vi "Teleop.vi"(10 "Match Info":T1={"Autonomous Elapsed Seconds"=0.0, "TeleOp Elapsed Seconds"=0.0, "Disabled Elapsed Seconds"=0.0, "Visited Autonomous"=FALSE, "Visited TeleOp"=FALSE, "Visited Disabled"=FALSE, "Autonomous Settings"={"Autonomous Style"=enum."Independent", "VI Refnum"=refnum}}, 11 "Call Context":T2) -> ()   [LabVIEW 2018]
doc: "This VI is called for each enabled TeleOp packet received from the DS. It is typically used to read from joysticks and other inputs and update I/O or setpoints for timed control loops. It should complete and return within 20 milliseconds or risk missing DS packets."
uses:
  <vilib>/Rock Robotics/WPI/DriverStation/WPI_DriverStationDerivedRobotMode.ctl
  <vilib>/Rock Robotics/WPI/DriverStation/WPI_DriverStationMatch Info.ctl
  <vilib>/Rock Robotics/WPI/ThirdParty/Phoenix-LabVIEW/Motor Controller/Controls/CTRE_Phoenix_MotorControl_ControlMode.ctl
  2fc8d68a-f7f1-41dc-b85b-aa47af0e09c4.vi
  <vilib>/Rock Robotics/WPI/Utilities/WPI_GetSetVariantRefNum.vi
  <vilib>/Rock Robotics/Network Tables/NT Write Boolean.vi
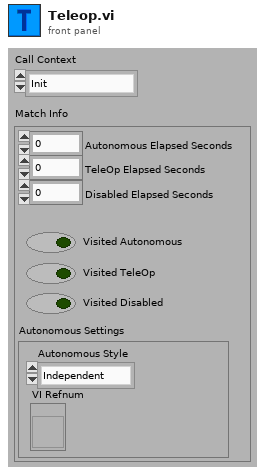
[diagram p1: front panel]
types:
  T1 = typedef "WPI_DriverStationMatch Info.ctl" = cluster{"Autonomous Elapsed Seconds":dbl, "TeleOp Elapsed Seconds":dbl, "Disabled Elapsed Seconds":dbl, "Visited Autonomous":bool, "Visited TeleOp":bool, "Visited Disabled":bool, "Autonomous Settings":cluster{"Autonomous Style":enum16{"Iterative", "Independent"}, "VI Refnum":refnum<vi>}}
  T2 = typedef "WPI_DriverStationDerivedRobotMode.ctl" = enum16{"Init", "Execute", "Stop"}
  T3 = enum16{"Low Ball", "Middle Ball", "High Ball", "High Hatch", "Middle Hatch", "Low Hatch", "Cargo Ball", "Ball Loading Station", "Ball Ground", "Reserve"}
  T4 = typedef "WPI_JoystickDevRef.ctl" = cluster{"Device":T5}
  T5 = typedef "WPI_JoystickDeviceEnum.ctl" = enum16{"USB 0", "USB 1", "USB 2", "USB 3", "USB 4", "USB 5"}
  T6 = cluster{"POVs[0]":i16, "POVs[1]":i16, "POVs[2]":i16, "POVs[3]":i16, "POVs[4]":i16, "POVs[5]":i16, "POVs[6]":i16, "POVs[7]":i16, "POVs[8]":i16}
  T7 = typedef "WPI_MotorControlDeviceRef.ctl" = cluster{"DeviceStatus":errorcluster, "Type":T8, "PWM":cluster{"PWM Channel":T9, "DeadBand":T10}, "CAN":cluster{"Device Number":u8, "SetOutput VI Ref":variant, "GetOutput VI Ref":variant, "Enable VI Ref":variant, "Disable VI Ref":variant, "Data":variant}, "Invert":bool, "DIO PWM":cluster{"PWM \"Enable\" Channel":T9, "DIOChannel":T11, "PWM Rate":dbl}}
  T8 = typedef "WPI_MotorControlType.ctl" = enum16{"PWM", "CAN", "DIO PWM"}
  T9 = typedef "FPGA_DIOPWMChannel.ctl" = enum8{"PWM 0", "PWM 1", "PWM 2", "PWM 3", "PWM 4", "PWM 5", "PWM 6", "PWM 7", "PWM 8", "PWM 9", "PWM MXP 0", "PWM MXP 1", "PWM MXP 2", "PWM MXP 3", "PWM MXP 4", "PWM MXP 5", "PWM MXP 6", "PWM MXP 7", "PWM MXP 8", "PWM MXP 9", "Invalid"}
  T10 = typedef "WPI_PWMDeadband.ctl" = cluster{"Name":string, "maxPositivePwm":i32, "minPositivePwm":i32, "centerPwm":i32, "maxNegativePwm":i32, "minNegativePwm":i32, "angularRange":u16}
  T11 = typedef "FPGA_DIOChannel.ctl" = enum8{"DIO 0", "DIO 1", "DIO 2", "DIO 3", "DIO 4", "DIO 5", "DIO 6", "DIO 7", "DIO 8", "DIO 9", "DIO MXP 0", "DIO MXP 1", "DIO MXP 2", "DIO MXP 3", "DIO MXP 4", "DIO MXP 5", "DIO MXP 6", "DIO MXP 7", "DIO MXP 8", "DIO MXP 9", "DIO MXP 10", "DIO MXP 11", "DIO MXP 12", "DIO MXP 13", "DIO MXP 14", "DIO MXP 15", "SPI Port CS1", "SPI Port CS2", "SPI Port CS3", "SPI Port MISO", "SPI Port MOSI", "Invalid"}
  T12 = typedef "CTRE_Phoenix_MotorControl_ControlMode.ctl" = u16
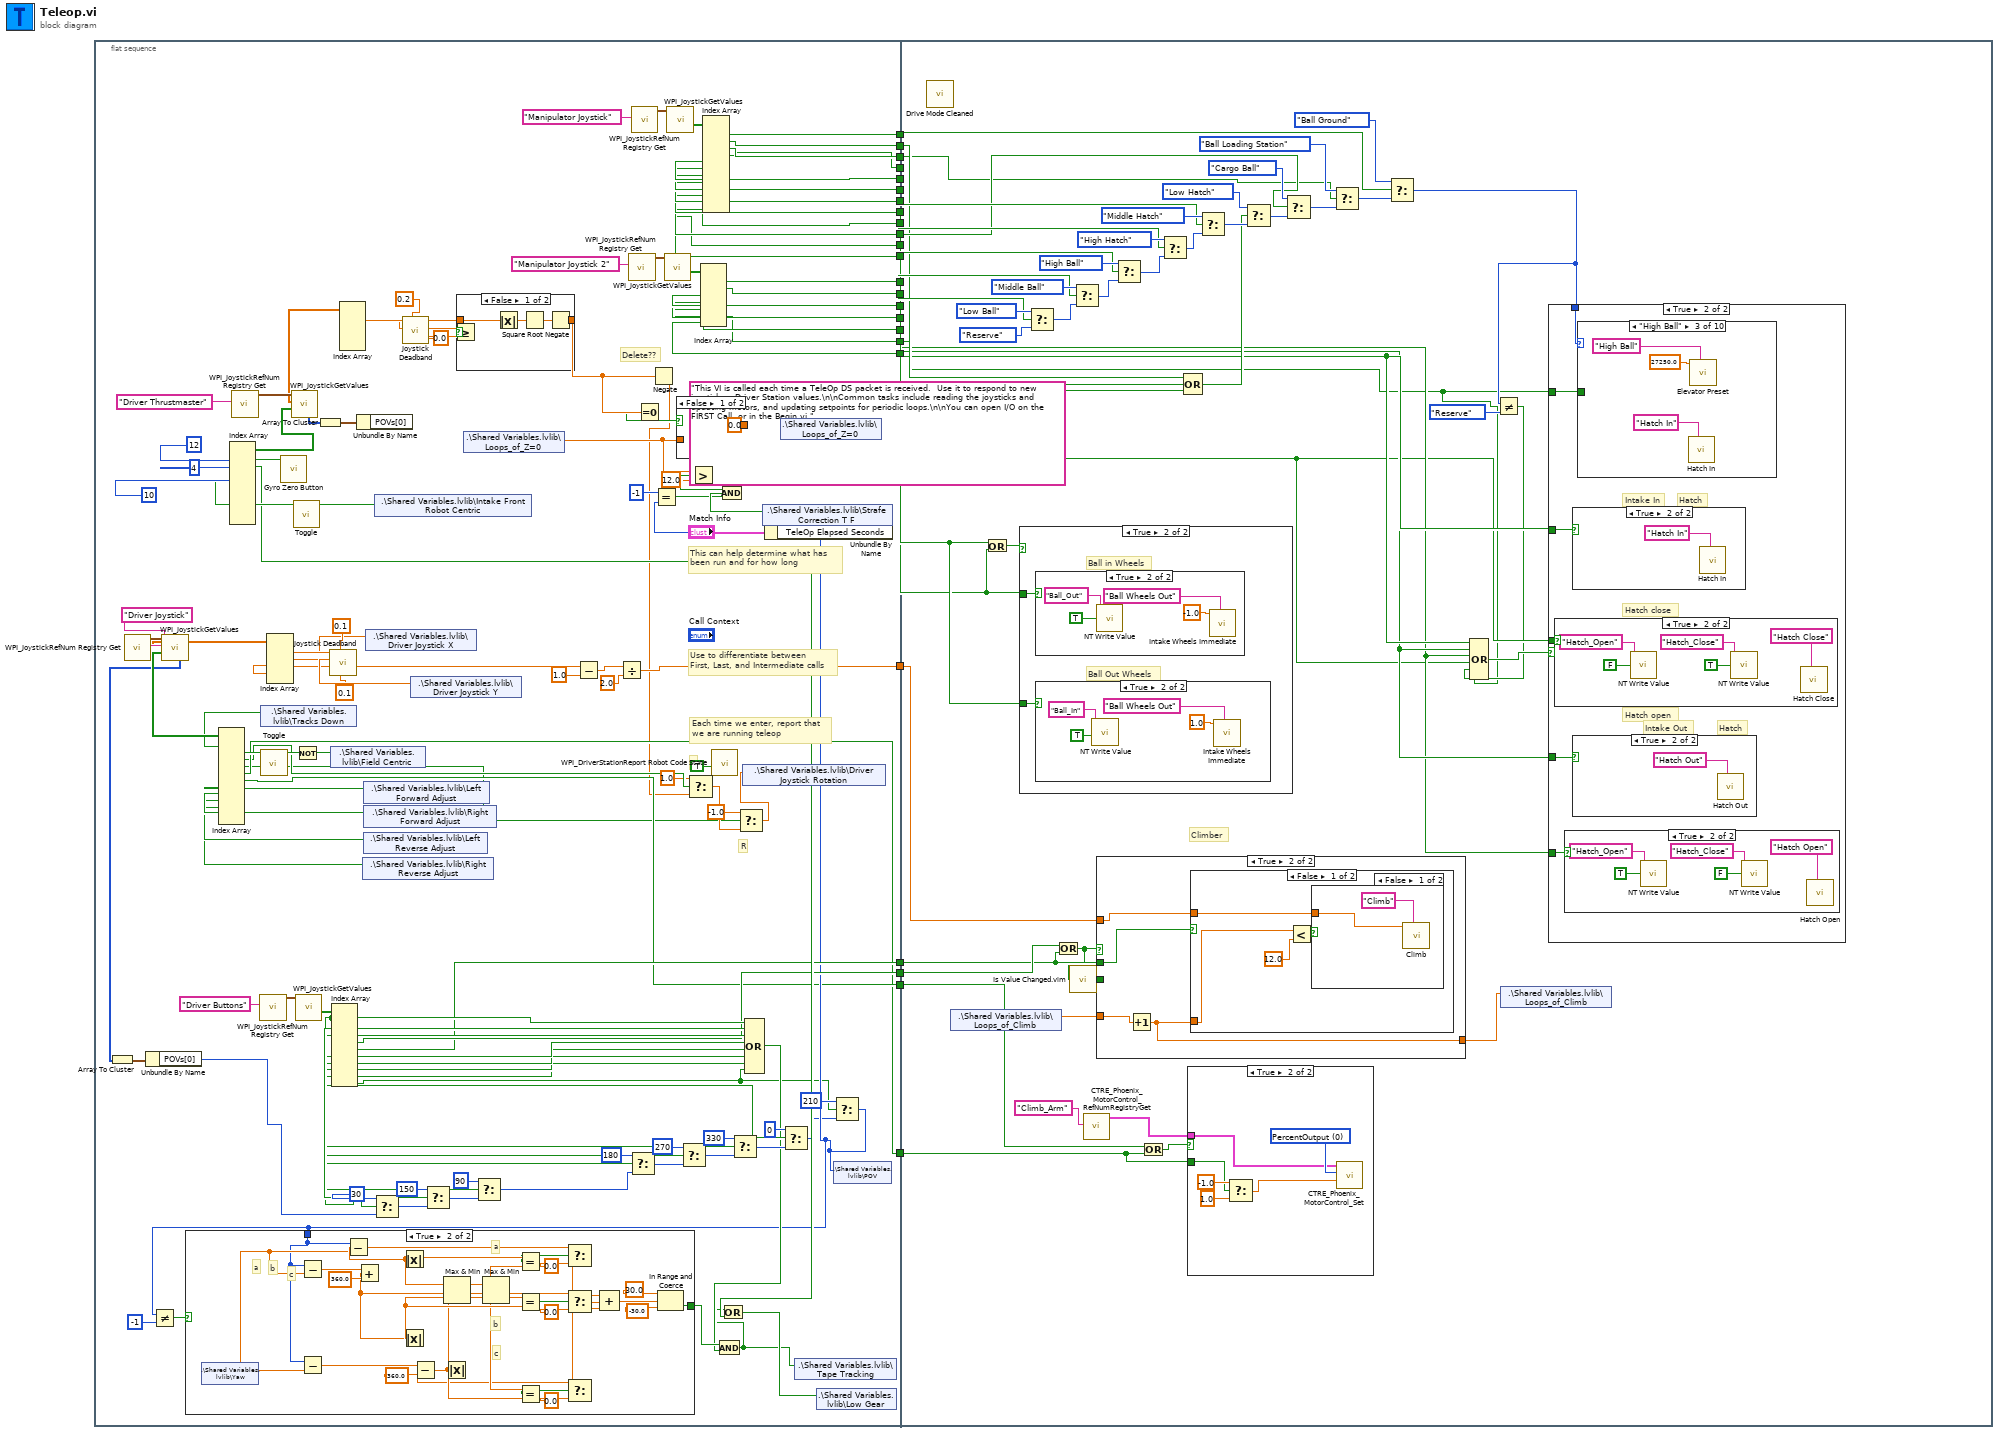
[diagram p0: block diagram]
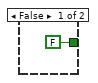
[diagram p2: hidden frame]
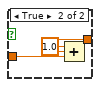
[diagram p3: hidden frame]
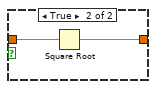
[diagram p4: hidden frame]
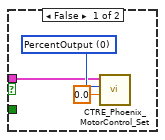
[diagram p5: hidden frame]
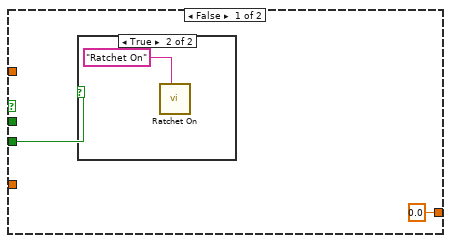
[diagram p6: hidden frame]
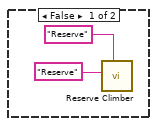
[diagram p7: hidden frame]
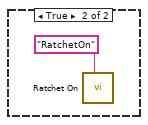
[diagram p8: hidden frame]
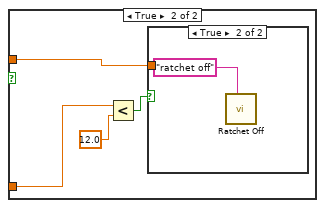
[diagram p9: hidden frame]
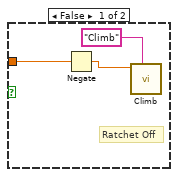
[diagram p10: hidden frame]
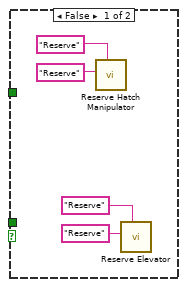
[diagram p11: hidden frame]
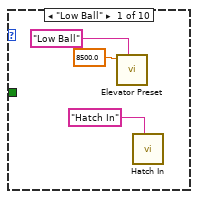
[diagram p12: hidden frame]
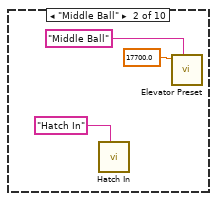
[diagram p13: hidden frame]
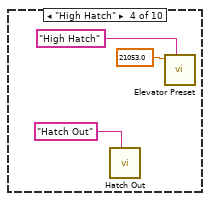
[diagram p14: hidden frame]
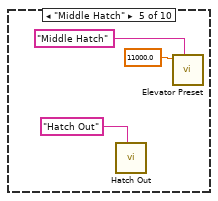
[diagram p15: hidden frame]
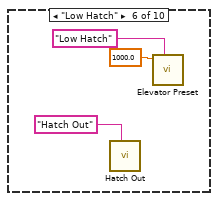
[diagram p16: hidden frame]
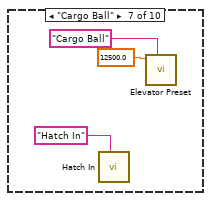
[diagram p17: hidden frame]
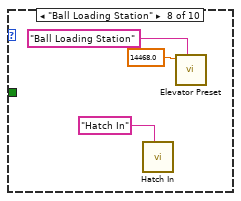
[diagram p18: hidden frame]
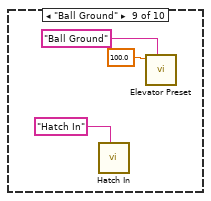
[diagram p19: hidden frame]
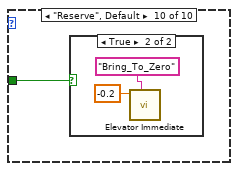
[diagram p20: hidden frame]
diagram:
  (unwired) "This VI is called each time a TeleOp DS packet is received.  Use it to respond to new joystick or Driver Station values.\n\nCommon tasks include reading the joysticks and updating motors, and updating setpoints for periodic loops.\n\nYou can open I/O on the FIRST Call, or in the Begin.vi."
  # "Each time we enter, report that\nwe are running teleop"
  # "Use to differentiate between\nFirst, Last, and Intermediate calls"
  # "This can help determine what has\nbeen run and for how long"
  n1 = flat-sequence {
    tunnel: [w50] -> w24
    tunnel: [w108] -> w23
    tunnel: [w107] -> w22
    tunnel: [w106] -> w21
    tunnel: [w105] -> w20
    tunnel: [w104] -> w19
    tunnel: [w103] -> w18
    tunnel: [w102] -> w17
    tunnel: [w101] -> w16
    tunnel: [w100] -> w15
    tunnel: [w99] -> w14
    tunnel: [w98] -> w13
    tunnel: [w97] -> w12
    tunnel: [w96] -> w11
    tunnel: [w95] -> w10
    tunnel: [w94] -> w9
    tunnel: [w93] -> w8
    tunnel: [w92] -> w7
    tunnel: [w91] -> w6
    tunnel: [w90] -> w5
    tunnel: [w53] -> w4
    tunnel: [w52] -> w3
    tunnel: [w36] -> w2
    tunnel: [w34] -> w1
    tunnel: w24 -> [w199]
    tunnel: w23 -> [w214]
    tunnel: w22 -> [w217]
    tunnel: w21 -> [w213]
    tunnel: w20 -> [w219]
    tunnel: w19 -> [w216]
    tunnel: w18 -> [w222]
    tunnel: w17 -> [w220]
    tunnel: w16 -> [w209]
    tunnel: w15 -> [w223]
    tunnel: w14 -> [w218]
    tunnel: w13 -> [w221]
    tunnel: w12 -> [w210]
    tunnel: w11 -> [w205]
    tunnel: w10 -> [_]
    tunnel: w9 -> [w208]
    tunnel: w8 -> [w206]
    tunnel: w7 -> [w207]
    tunnel: w6 -> [w197]
    tunnel: w5 -> [w212]
    tunnel: w4 -> [w201]
    tunnel: w3 -> [w200]
    tunnel: w2 -> [w193]
    tunnel: w1 -> [w192]
    frame #0 {
      # "R"
      # "L"
      # "Delete??"
      n2 = call <vilib>:"WPI_JoystickRefNum Registry Get.vi"("refnum name"="Driver Joystick") -> ("JoystickDevRef"=w149:T4)  [unwired: 1 in, 9 out]
      n3 = call <vilib>:"WPI_JoystickGetValues.vi"("JoystickDevRef"=w149) -> ("Buttons"=w135:bool[], "Axes"=w147:dbl[], "POVs"=w122:i16[])  [unwired: 6 in, 2 out]
      n4 = Array To Cluster(array=w122) -> (cluster=w123:T6)
      n5 = Unbundle By Name(w123) -> ("POVs[0]"=w35:i16)
      n6 = Index Array(array=w135) -> (element #1=w111:bool, element #2=w110:bool, element #3=w33:bool, element #4=w31:bool, element #5=w34:bool, element #6=w36:bool, element #7=w120:bool, element #8=w119:bool, element #9=w118:bool, element #10=w117:bool)  [unwired: 12 in, 2 out]
      n7 = call <vilib>:"WPI_JoystickRefNum Registry Get.vi"("refnum name"="Driver Thrustmaster") -> ("JoystickDevRef"=w137:T4)  [unwired: 9 in, 1 out]
      n8 = call <vilib>:"WPI_JoystickRefNum Registry Get.vi"("refnum name"="Driver Buttons") -> ("JoystickDevRef"=w88:T4)  [unwired: 1 in, 9 out]
      n9 = shared-variable ".\\Shared Variables.lvlib\\Tracks Down"(w111) -> ()  [unwired: 1 in, 1 out]
      n10 = call "Toggle.vi"("Input"=w110) -> ("Output"=w142:bool)  [unwired: 9 in, 1 out]
      n11 = Index Array(array=w147) -> (element #1=w141:dbl, element #2=w140:dbl, element #4=w112:dbl)  [unwired: 5 in, 2 out]
      n12 = call <vilib>:"WPI_JoystickGetValues.vi"("JoystickDevRef"=w137) -> ("Buttons"=w132:bool[], "Axes"=w136:dbl[], "POVs"=w124:i16[])  [unwired: 6 in, 2 out]
      n13 = Index Array(array=w132, index #1=12 ("index"), index #2=4 ("index"), index #4=10 ("index")) -> (element #1=w130:bool, element #2=w56:bool, element #4=w125:bool)  [unwired: 7 in, 7 out]
      n14 = call "Gyro Zero Button.vi"("Boolean"=w130) -> ()  [unwired: 11 in]
      n15 = call "Toggle.vi"("Input"=w125) -> ("Output"=w126:bool)  [unwired: 9 in, 1 out]
      n16 = Not(x=w142) -> (.not. x?=w139:bool)
      n17 = call <vilib>:"WPI_JoystickGetValues.vi"("JoystickDevRef"=w88) -> ("Buttons"=w48:bool[])  [unwired: 6 in, 4 out]
      n18 = Array To Cluster(array=w124) -> (cluster=w128:T6)
      n19 = call "Joystick Deadband.vi"("Z Deadband"=0.1, "X Y Deadband"=0.1, "Z"=w112, "Y"=w140, "X"=w141) -> ("Z Out"=w39:dbl, "Y Out"=w143:dbl, "X Out"=w116:dbl)  [unwired: 4 in]
      n20 = shared-variable ".\\Shared Variables.lvlib\\Field Centric"(w139) -> ()  [unwired: 1 in, 1 out]
      n21 = Index Array(array=w48) -> (element #1=w68:bool, element #2=w74:bool, element #3=w73:bool, element #4=w53:bool, element #5=w52:bool, element #6=w72:bool, element #7=w71:bool, element #8=w70:bool, element #9=w69:bool, element #10=w40:bool)  [unwired: 10 in]
      n22 = Index Array(array=w136) -> (element #1=w115:dbl)  [unwired: 5 in, 4 out]
      n23 = Unbundle By Name(w128) -> ()  [unwired: 1 out]
      n24 = shared-variable ".\\Shared Variables.lvlib\\Right Reverse Adjust"(w117) -> ()  [unwired: 1 in, 1 out]
      n25 = shared-variable ".\\Shared Variables.lvlib\\Left Forward Adjust"(w120) -> ()  [unwired: 1 in, 1 out]
      n26 = shared-variable ".\\Shared Variables.lvlib\\Right Forward Adjust"(w119) -> ()  [unwired: 1 in, 1 out]
      n27 = shared-variable ".\\Shared Variables.lvlib\\Left Reverse Adjust"(w118) -> ()  [unwired: 1 in, 1 out]
      n28 = shared-variable ".\\Shared Variables.lvlib\\Driver Joystick X"(w116) -> ()  [unwired: 1 in, 1 out]
      n29 = Select(t=i16 30, s=w68, f=w35) -> (s? t:f=w82:i16)
      n30 = shared-variable ".\\Shared Variables.lvlib\\Intake Front Robot Centric"(w126) -> ()  [unwired: 1 in, 1 out]
      n31 = call "Joystick Deadband.vi"("X Y Deadband"=0.2, "X"=w115) -> ("X Out"=w113:dbl)  [unwired: 7 in, 2 out]
      n32 = shared-variable ".\\Shared Variables.lvlib\\Driver Joystick Y"(w143) -> ()  [unwired: 1 in, 1 out]
      n33 = Select(t=i16 150, s=w74, f=w82) -> (s? t:f=w81:i16)
      n34 = Greater Or Equal?(x=w113, y=0.0) -> (x >= y?=w134:bool)
      n35 = case shown="False" w134 {
        tunnel: [w183 w187] -> w64
        tunnel: w113 -> [w182 w186]
        frame False {
          n36 = Absolute Value(x=w182) -> (abs(x)=w185:dbl)
          n37 = Square Root(x=w185) -> (sqrt(x)=w184:dbl)
          n38 = Negate(x=w184) -> (-x=w183:dbl)
        }
        frame True {
          n39 = Square Root(x=w186) -> (sqrt(x)=w187:dbl)
        }
      }
      n40 = shared-variable ".\\Shared Variables.lvlib\\Loops_of_Z=0"() -> (w60:dbl)  [unwired: 1 in, 1 out]
      n41 = Select(t=i16 90, s=w73, f=w81) -> (s? t:f=w49:i16)
      n42 = Subtract(x=w39, y=1.0) -> (x-y=w38:dbl)
      n43 = Divide(x=w38, y=2.0) -> (x/y=w50:dbl)
      n44 = call <vilib>:"WPI_JoystickRefNum Registry Get.vi"("refnum name"="Manipulator Joystick 2") -> ("JoystickDevRef"=w89:T4)  [unwired: 1 in, 9 out]
      n45 = Select(t=i16 180, s=w72, f=w49) -> (s? t:f=w79:i16)
      n46 = call <vilib>:"WPI_JoystickRefNum Registry Get.vi"("refnum name"="Manipulator Joystick") -> ("JoystickDevRef"=w145:T4)  [unwired: 1 in, 9 out]
      n47 = Equal To 0?(x=w64) -> (x = 0?=w63:bool)
      n48 = Negate(x=w64) -> (-x=w28:dbl)
      n49 = call <vilib>:"WPI_JoystickGetValues.vi"("JoystickDevRef"=w89) -> ("Buttons"=w46:bool[])  [unwired: 6 in, 4 out]
      n50 = call <vilib>:"WPI_JoystickGetValues.vi"("JoystickDevRef"=w145) -> ("Buttons"=w47:bool[])  [unwired: 6 in, 4 out]
      n51 = case shown="False" w63 {
        tunnel: w60 -> [_ w181]
        tunnel: [0.0 w179] -> w62
        frame False {
        }
        frame True {
          n52 = Add(x=1.0, y=w181) -> (x+y=w179:dbl)
        }
      }
      n53 = Select(t=i16 270, s=w71, f=w79) -> (s? t:f=w77:i16)
      n54 = Select(t=1.0, s=w33, f=w28) -> (s? t:f=w32:dbl)
      n55 = Greater?(x=w60, y=12.0) -> (0:w61:bool)
      n56 = Index Array(array=w46) -> (element #1=w96:bool, element #2=w95:bool, element #3=w94:bool, element #4=w93:bool, element #5=w92:bool, element #6=w91:bool, element #7=w90:bool)  [unwired: 7 in]
      n57 = Index Array(array=w47) -> (element #1=w108:bool, element #2=w107:bool, element #3=w106:bool, element #4=w105:bool, element #5=w104:bool, element #6=w103:bool, element #7=w102:bool, element #8=w101:bool, element #9=w100:bool, element #10=w99:bool, element #11=w98:bool, element #12=w97:bool)  [unwired: 12 in]
      n58 = Select(t=i16 330, s=w70, f=w77) -> (s? t:f=w75:i16)
      n59 = Select(t=-1.0, s=w31, f=w32) -> (s? t:f=w27:dbl)
      n60 = shared-variable ".\\Shared Variables.lvlib\\Driver Joystick Rotation"(w27) -> ()  [unwired: 1 in, 1 out]
      n61 = Compound Arithmetic op=OR(w68, w74, w73, w72, w71, w70, w69, w40) -> (w57:bool)
      n62 = shared-variable ".\\Shared Variables.lvlib\\Loops_of_Z=0"(w62) -> ()  [unwired: 1 in, 1 out]
      n63 = Select(t=i16 0, s=w69, f=w75) -> (s? t:f=w42:i16)
      n64 = Select(t=i16 210, s=w40, f=w42) -> (s? t:f=w43:i16)
      n65 = Not Equal?(x=w43, y=i16 -1) -> (x != y?=w45:bool)
      n66 = case shown="True" w45 {
        tunnel: [FALSE w175] -> w58
        tunnel: w43 -> [_ w152]
        frame False {
        }
        frame True {
          # "c"
          # "b"
          # "a"
          # "c"
          # "b"
          # "a"
          n67 = shared-variable ".\\Shared Variables.lvlib\\Yaw"() -> (w153:dbl)  [unwired: 1 in, 1 out]
          n68 = Subtract(x=w152, y=w153) -> (x-y=w174:dbl)
          n69 = Subtract(x=w152, y=w153) -> (x-y=w172:dbl)
          n70 = Subtract(x=w152, y=w153) -> (x-y=w163:dbl)
          n71 = Add(x=w174, y=360.0) -> (x+y=w164:dbl)
          n72 = Absolute Value(x=w163) -> (abs(x)=w169:dbl)
          n73 = Absolute Value(x=w164) -> (abs(x)=w168:dbl)
          n74 = Subtract(x=w172, y=360.0) -> (x-y=w162:dbl)
          n75 = Max & Min(x=w169, y=w168) -> (min(x,y)=w170:dbl)  [unwired: 1 out]
          n76 = Absolute Value(x=w162) -> (abs(x)=w166:dbl)
          n77 = Max & Min(x=w170, y=w166) -> (min(x,y)=w167:dbl)  [unwired: 1 out]
          n78 = Equal?(x=w169, y=w167) -> (x = y?=w161:bool)
          n79 = Equal?(x=w167, y=w168) -> (x = y?=w165:bool)
          n80 = Equal?(x=w167, y=w166) -> (x = y?=w160:bool)
          n81 = Select(t=w163, s=w161, f=0.0) -> (s? t:f=w156:dbl)
          n82 = Select(t=w164, s=w165, f=0.0) -> (s? t:f=w155:dbl)
          n83 = Select(t=w162, s=w160, f=0.0) -> (s? t:f=w154:dbl)
          n84 = Compound Arithmetic op=ADD(w156, w155, w154) -> (w151:dbl)
          n85 = In Range and Coerce(upper limit=30.0, x=w151, lower limit=-30.0) -> (In Range?=w175:bool)  [unwired: 1 out]
        }
      }
      n86 = Equal?(x=i16 -1, y=w43) -> (x = y?=w65:bool)
      n87 = And(x=w61, y=w65) -> (x .and. y?=w66:bool)
      n88 = Compound Arithmetic op=AND(w58, w57) -> (w54:bool)
      n89 = Or(x=w54, y=w56) -> (x .or. y?=w55:bool)
      n90 = shared-variable ".\\Shared Variables.lvlib\\Strafe Correction T F"(w66) -> ()  [unwired: 1 in, 1 out]
      n91 = shared-variable ".\\Shared Variables.lvlib\\Tape Tracking"(w54) -> ()  [unwired: 1 in, 1 out]
      n92 = shared-variable ".\\Shared Variables.lvlib\\Low Gear"(w55) -> ()  [unwired: 1 in, 1 out]
      n93 = shared-variable ".\\Shared Variables.lvlib\\POV"(w43) -> ()  [unwired: 1 in, 1 out]
    }
    frame #1 {
      # "Climber"
      n94 = call "Drive Mode Cleaned.vi"() -> ()  [unwired: 12 in]
      n95 = shared-variable ".\\Shared Variables.lvlib\\Loops_of_Climb"() -> (w189:dbl)  [unwired: 1 in, 1 out]
      n96 = Or(x=w210, y=w209) -> (x .or. y?=w211:bool)
      n97 = case shown="True" w211 {
        tunnel: w210 -> [_ w336]
        tunnel: w209 -> [_ w335]
        frame False {
          n98 = call-poly <vilib>:"NT Write Value.vi"("Boolean"=FALSE, "Name"="Ball_Out") -> ()  [unwired: 9 in, 1 out]
          n99 = call "Reserve Intake.vi"("Description"="Reserve", "Command Name"="Reserve") -> ()  [unwired: 9 in, 1 out]
          n100 = call-poly <vilib>:"NT Write Value.vi"("Boolean"=FALSE, "Name"="Ball_In") -> ()  [unwired: 9 in, 1 out]
        }
        frame True {
          # "Ball in Wheels"
          # "Ball Out Wheels"
          n101 = case shown="True" w335 {
            frame False {
            }
            frame True {
              n102 = call-poly <vilib>:"NT Write Value.vi"("Boolean"=TRUE, "Name"="Ball_Out") -> ()  [unwired: 9 in, 1 out]
              n103 = call "Intake Wheels Immediate.vi"("Description"="Ball Wheels Out", "Setpoint"=-1.0) -> ()  [unwired: 9 in, 1 out]
            }
          }
          n104 = case shown="True" w336 {
            frame False {
            }
            frame True {
              n105 = call-poly <vilib>:"NT Write Value.vi"("Boolean"=TRUE, "Name"="Ball_In") -> ()  [unwired: 9 in, 1 out]
              n106 = call "Intake Wheels Immediate.vi"("Description"="Ball Wheels Out", "Setpoint"=1.0) -> ()  [unwired: 9 in, 1 out]
            }
          }
        }
      }
      n107 = Select(t=T3."Low Ball" ("Enum"), s=w219, f=T3."Reserve" ("Enum")) -> (s? t:f=w241:T3)
      n108 = Or(x=w201, y=w200) -> (x .or. y?=w191:bool)
      n109 = call "Is Value Changed.vim"("value"=w191) -> ("changed or first call?"=w190:bool)
      n110 = Select(t=T3."Middle Ball" ("Enum"), s=w220, f=w241) -> (s? t:f=w240:T3)
      n111 = call <vilib>:"CTRE_Phoenix_MotorControl_RefNumRegistryGet.vi"("refnum name"="Climb_Arm") -> ("PhoenixMotorControlDevRef"=w195:T7)  [unwired: 9 in, 1 out]
      n112 = case shown="True" w191 {
        tunnel: w200 -> [_ w259]
        tunnel: w199 -> [_ w258]
        tunnel: w190 -> [w252 _]
        tunnel: w189 -> [_ w257]
        tunnel: [0.0 w256] -> w188
        frame False {
          n113 = case shown="True" w252 {
            frame False {
              n114 = call "Reserve Climber.vi"("Description"="Reserve", "Command Name"="Reserve" ("Description")) -> ()  [unwired: 9 in, 1 out]
            }
            frame True {
              n115 = call "Ratchet On.vi"("Description"="Ratchet On") -> ()  [unwired: 10 in, 1 out]
            }
          }
        }
        frame True {
          n116 = Increment(x=w257) -> (x+1=w256:dbl)
          n117 = case shown="False" w259 {
            tunnel: w258 -> [w263 w270]
            tunnel: w256 -> [w260 w267]
            frame False {
              n118 = Less?(x=w260, y=12.0 ("x")) -> (x < y?=w262:bool)
              n119 = case shown="False" w262 {
                tunnel: w263 -> [w264 _]
                frame False {
                  n120 = call "Climb.vi"("Description"="Climb", "Setpoint"=w264) -> ()  [unwired: 9 in, 1 out]
                }
                frame True {
                  n121 = call "Ratchet On.vi"("Description"="RatchetOn") -> ()  [unwired: 10 in, 1 out]
                }
              }
            }
            frame True {
              n122 = Less?(x=w267, y=12.0 ("x")) -> (x < y?=w268:bool)
              n123 = case shown="True" w268 {
                tunnel: w270 -> [w272 _]
                frame False {
                  # "Ratchet Off"
                  n124 = Negate(x=w272) -> (-x=w271:dbl)
                  n125 = call "Climb.vi"("Description"="Climb", "Setpoint"=w271) -> ()  [unwired: 9 in, 1 out]
                }
                frame True {
                  n126 = call "Ratchet Off.vi"("Description"="ratchet off") -> ()  [unwired: 10 in, 1 out]
                }
              }
            }
          }
        }
      }
      n127 = Select(t=T3."High Ball" ("Enum"), s=w221, f=w240) -> (s? t:f=w239:T3)
      n128 = Or(x=w193, y=w192) -> (x .or. y?=w194:bool)
      n129 = Select(t=T3."High Hatch" ("Enum"), s=w223, f=w239) -> (s? t:f=w238:T3)
      n130 = Compound Arithmetic op=OR(w217, w216, w212) -> (w215:bool)
      n131 = case shown="True" w194 {
        tunnel: w195 -> [w242 w245]
        tunnel: w192 -> [_ w247]
        frame False {
          w244 = T12 0 items=["PercentOutput"=0, "Position"=1, "Velocity"=2, "Current"=3, "Follower"=5, "MotionProfile"=6, "MotionMagic"=7, "MotionProfileArc"=10, "Disabled"=15] ("Control Mode")
          n132 = call <vilib>:"CTRE_Phoenix_MotorControl_Set.vi"("Output"=0.0, "Control Mode"=w244, "PhoenixMotorControlDevRef"=w242) -> ()  [unwired: 7 in, 2 out]
        }
        frame True {
          w250 = T12 0 items=["PercentOutput"=0, "Position"=1, "Velocity"=2, "Current"=3, "Follower"=5, "MotionProfile"=6, "MotionMagic"=7, "MotionProfileArc"=10, "Disabled"=15] ("Control Mode")
          n133 = Select(t=-1.0, s=w247, f=1.0) -> (s? t:f=w246:dbl)
          n134 = call <vilib>:"CTRE_Phoenix_MotorControl_Set.vi"("Output"=w246, "Control Mode"=w250, "PhoenixMotorControlDevRef"=w245) -> ()  [unwired: 7 in, 2 out]
        }
      }
      n135 = Select(t=T3."Middle Hatch" ("Enum"), s=w222, f=w238) -> (s? t:f=w237:T3)
      n136 = Select(t=T3."Low Hatch" ("Enum"), s=w215, f=w237) -> (s? t:f=w236:T3)
      n137 = Select(t=T3."Cargo Ball" ("Enum"), s=w218, f=w236) -> (s? t:f=w235:T3)
      n138 = Select(t=T3."Ball Loading Station" ("Enum"), s=w213, f=w235) -> (s? t:f=w225:T3)
      n139 = Select(t=T3."Ball Ground" ("Enum"), s=w214, f=w225) -> (s? t:f=w203:T3)
      n140 = Not Equal?(x=w203, y=T3."Reserve" ("Enum")) -> (x != y?=w198:bool)
      n141 = Compound Arithmetic op=OR(w208, w207, w206, w205, w198, w197) -> (w204:bool)
      n142 = shared-variable ".\\Shared Variables.lvlib\\Loops_of_Climb"(w188) -> ()  [unwired: 1 in, 1 out]
      n143 = case shown="True" w204 {
        tunnel: w208 -> [_ w284]
        tunnel: w206 -> [_ w283]
        tunnel: w207 -> [_ w282]
        tunnel: w205 -> [_ w281]
        tunnel: w203 -> [_ w280]
        tunnel: w197 -> [_ w279]
        frame False {
          n144 = call "Reserve Hatch Manipulator.vi"("Description"="Reserve", "Command Name"="Reserve") -> ()  [unwired: 9 in, 1 out]
          n145 = call "Reserve Elevator.vi"("Description"="Reserve", "Command Name"="Reserve") -> ()  [unwired: 9 in, 1 out]
        }
        frame True {
          # "Hatch"
          # "Hatch"
          # "Hatch open"
          # "Hatch close"
          # "Intake In"
          # "Intake Out"
          n146 = case shown="True" w281 {
            frame False {
            }
            frame True {
              n147 = call-poly <vilib>:"NT Write Value.vi"("Boolean"=FALSE, "Name"="Hatch_Open") -> ()  [unwired: 9 in, 1 out]
              n148 = call-poly <vilib>:"NT Write Value.vi"("Boolean"=TRUE, "Name"="Hatch_Close") -> ()  [unwired: 9 in, 1 out]
              n149 = call "Hatch Close.vi"("Description"="Hatch Close") -> ()  [unwired: 10 in, 1 out]
            }
          }
          n150 = case shown="True" w283 {
            frame False {
            }
            frame True {
              n151 = call-poly <vilib>:"NT Write Value.vi"("Boolean"=TRUE, "Name"="Hatch_Open") -> ()  [unwired: 9 in, 1 out]
              n152 = call-poly <vilib>:"NT Write Value.vi"("Boolean"=FALSE, "Name"="Hatch_Close") -> ()  [unwired: 9 in, 1 out]
              n153 = call "Hatch Open.vi"("Description"="Hatch Open") -> ()  [unwired: 10 in, 1 out]
            }
          }
          n154 = case shown="True" w284 {
            frame False {
            }
            frame True {
              n155 = call "Hatch In.vi"("Description"="Hatch In") -> ()  [unwired: 10 in, 1 out]
            }
          }
          n156 = case shown="True" w282 {
            frame False {
            }
            frame True {
              n157 = call "Hatch Out.vi"("Description"="Hatch Out") -> ()  [unwired: 10 in, 1 out]
            }
          }
          n158 = case shown="\"High Ball\"" w280 {
            tunnel: w279 -> [_ _ _ _ _ _ _ _ _ w312]
            frame "Low Ball" {
              n159 = call "Elevator Preset.vi"("Description"="Low Ball", "Position"=8500.0) -> ()  [unwired: 9 in, 1 out]
              n160 = call "Hatch In.vi"("Description"="Hatch In") -> ()  [unwired: 10 in, 1 out]
            }
            frame "Middle Ball" {
              n161 = call "Hatch In.vi"("Description"="Hatch In") -> ()  [unwired: 10 in, 1 out]
              n162 = call "Elevator Preset.vi"("Description"="Middle Ball", "Position"=17700.0) -> ()  [unwired: 9 in, 1 out]
            }
            frame "High Ball" {
              n163 = call "Hatch In.vi"("Description"="Hatch In") -> ()  [unwired: 10 in, 1 out]
              n164 = call "Elevator Preset.vi"("Description"="High Ball", "Position"=27250.0) -> ()  [unwired: 9 in, 1 out]
            }
            frame "High Hatch" {
              n165 = call "Hatch Out.vi"("Description"="Hatch Out") -> ()  [unwired: 10 in, 1 out]
              n166 = call "Elevator Preset.vi"("Description"="High Hatch", "Position"=21053.0) -> ()  [unwired: 9 in, 1 out]
            }
            frame "Middle Hatch" {
              n167 = call "Hatch Out.vi"("Description"="Hatch Out") -> ()  [unwired: 10 in, 1 out]
              n168 = call "Elevator Preset.vi"("Description"="Middle Hatch", "Position"=11000.0) -> ()  [unwired: 9 in, 1 out]
            }
            frame "Low Hatch" {
              n169 = call "Hatch Out.vi"("Description"="Hatch Out") -> ()  [unwired: 10 in, 1 out]
              n170 = call "Elevator Preset.vi"("Description"="Low Hatch", "Position"=1000.0) -> ()  [unwired: 9 in, 1 out]
            }
            frame "Cargo Ball" {
              n171 = call "Hatch In.vi"("Description"="Hatch In") -> ()  [unwired: 10 in, 1 out]
              n172 = call "Elevator Preset.vi"("Description"="Cargo Ball", "Position"=12500.0) -> ()  [unwired: 9 in, 1 out]
            }
            frame "Ball Loading Station" {
              n173 = call "Hatch In.vi"("Description"="Hatch In") -> ()  [unwired: 10 in, 1 out]
              n174 = call "Elevator Preset.vi"("Description"="Ball Loading Station", "Position"=14468.0) -> ()  [unwired: 9 in, 1 out]
            }
            frame "Ball Ground" {
              n175 = call "Hatch In.vi"("Description"="Hatch In") -> ()  [unwired: 10 in, 1 out]
              n176 = call "Elevator Preset.vi"("Description"="Ball Ground", "Position"=100.0) -> ()  [unwired: 9 in, 1 out]
            }
            frame "Reserve", Default {
              n177 = case shown="True" w312 {
                frame False {
                  n178 = call "Reserve Elevator.vi"("Description"="Reserve", "Command Name"="Reserve") -> ()  [unwired: 9 in, 1 out]
                }
                frame True {
                  n179 = call "Elevator Immediate.vi"("Description"="Bring_To_Zero", "Speed"=-0.2) -> ()  [unwired: 9 in, 1 out]
                }
              }
            }
          }
        }
      }
    }
  }
  n180 = call <vilib>:"WPI_DriverStationReport Robot Code State.vi"("TeleOp"=TRUE ("Autonomous")) -> ()  [unwired: 10 in, 1 out]
  n181 = Unbundle By Name("Match Info") -> ()  [unwired: 1 out]
